vi "Default Config VI.vi"(8 "error in (no error)":errorcluster, 11 "Plugin in":refnum<class "Plugin.lvclass">) -> (0 "error out":errorcluster, 3 "Plugin out":refnum<class "Plugin.lvclass">)   [LabVIEW 2015, in "Plugin.lvclass"]
uses:
  Plugin.lvclass
panel:
  out "MSG":string
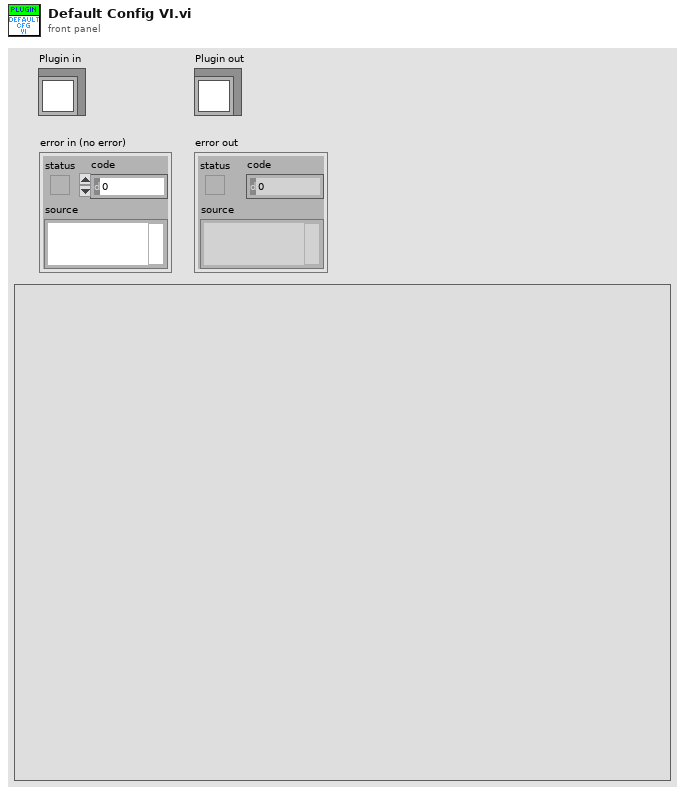
[diagram p1: front panel]
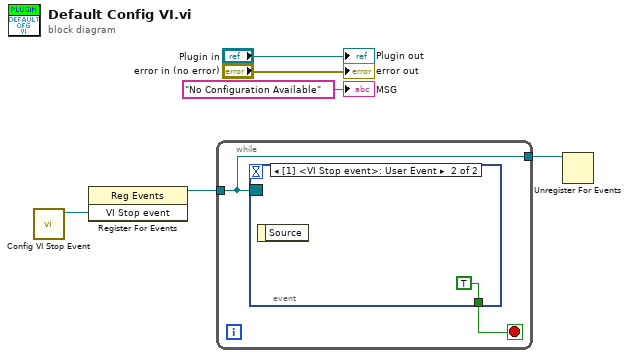
[diagram p0: block diagram]
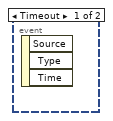
[diagram p2: hidden frame]
diagram:
  n1 = call "Config VI Stop Event.vi"() -> ("VI Stop event"=w4:refnum<user-event>)  [unwired: 11 in]
  n2 = register-events(w4) -> (reference out=w3:refnum<event-registration>)  [unwired: 2 in, 1 out]
  n3 = while {
    tunnel: w3 -> [w7]
    tunnel: [w7] -> w2
    stop <- w8 stop-if-true
    n4 = event shown="[1] <VI Stop event>: User Event" {
      selector: w7 -> [_ _]
      dyn-events: _ -> [_ _]
      timeout: _ -> [_ _]
      tunnel: [_ TRUE] -> w8
      event Timeout {
        n5 = event-data() -> ()  [unwired: 1 in, 3 out]
      }
      event User Event {
        n6 = event-data() -> ()  [unwired: 1 in, 1 out]
      }
    }
  }
  n7 = Unregister For Events(event registration refnum=w2) -> ()  [unwired: 1 in, 1 out]
  "error out" <- "error in (no error)"
  "Plugin out" <- "Plugin in"
  "MSG" <- "No Configuration Available" ("MSG")
